vi "raw stick values to [-1.0, 1.0].vi"(4 "Max controller reading":dbl=29767.0, 5 "Deadband value (0)":i32, 6 "deadband limit":i32=3000, 7 "Reverse y-axis?":bool=TRUE, 8 "Reverse x-axis?":bool=TRUE, 9 "raw y-axis":i32, 10 "raw x-axis":i32) -> (2 "normalized y-axis":dbl, 3 "normalized x-axis":dbl)   [LabVIEW 2018]
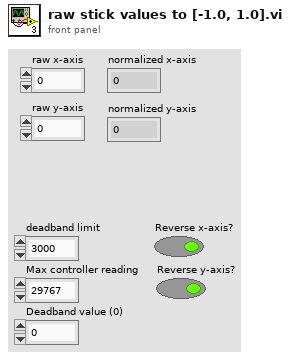
[diagram p1: front panel]
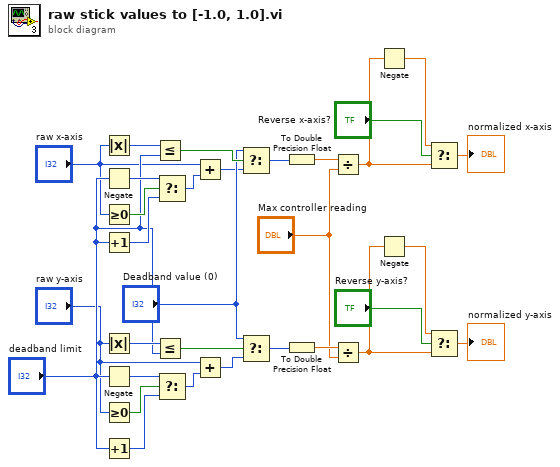
[diagram p0: block diagram]
diagram:
  n1 = Absolute Value(x="raw x-axis") -> (abs(x)=w28:i32)
  n2 = Negate(x="deadband limit") -> (-x=w15:i32)
  n3 = Greater Or Equal To 0?(x="raw x-axis") -> (x >= 0?=w24:bool)
  n4 = Increment(x="deadband limit") -> (x+1=w14:i32)
  n5 = Absolute Value(x="raw y-axis") -> (abs(x)=w27:i32)
  n6 = Negate(x="deadband limit") -> (-x=w13:i32)
  n7 = Greater Or Equal To 0?(x="raw y-axis") -> (x >= 0?=w22:bool)
  n8 = Increment(x="deadband limit") -> (x+1=w12:i32)
  n9 = Less Or Equal?(x=w28, y="deadband limit") -> (x <= y?=w30:bool)
  n10 = Less Or Equal?(x=w27, y="deadband limit") -> (x <= y?=w31:bool)
  n11 = Select(t=w15, s=w24, f=w14) -> (s? t:f=w23:i32)
  n12 = Select(t=w13, s=w22, f=w12) -> (s? t:f=w21:i32)
  n13 = Add(x="raw x-axis", y=w23) -> (x+y=w26:i32)
  n14 = Add(x="raw y-axis", y=w21) -> (x+y=w25:i32)
  n15 = Select(t="Deadband value (0)", s=w30, f=w26) -> (s? t:f=w20:i32)
  n16 = Select(t="Deadband value (0)", s=w31, f=w25) -> (s? t:f=w19:i32)
  n17 = To Double Precision Float(number=w20) -> (double precision float=w18:dbl)
  n18 = To Double Precision Float(number=w19) -> (double precision float=w17:dbl)
  n19 = Divide(x=w18, y="Max controller reading") -> (x/y=w8:dbl)
  n20 = Divide(x=w17, y="Max controller reading") -> (x/y=w6:dbl)
  n21 = Negate(x=w8) -> (-x=w7:dbl)
  n22 = Negate(x=w6) -> (-x=w5:dbl)
  n23 = Select(t=w7, s="Reverse x-axis?", f=w8) -> (s? t:f=→"normalized x-axis":dbl)
  n24 = Select(t=w5, s="Reverse y-axis?", f=w6) -> (s? t:f=→"normalized y-axis":dbl)
